vi "aryth_mux.vi"(2 "C":T1, 3 "A-B":bool, 4 "A+B":cluster{"S":bool, "C":bool}) -> (0 "R":bool, 1 "S1":bool)   [LabVIEW 2013]
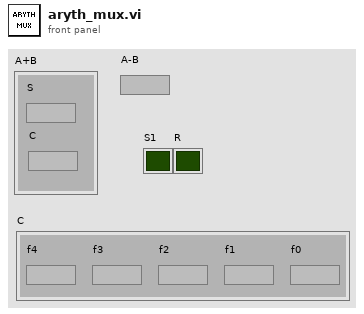
[diagram p1: front panel]
types:
  T1 = cluster{"f4":bool, "f3":bool, "f2":bool, "f1":bool, "f0":bool}
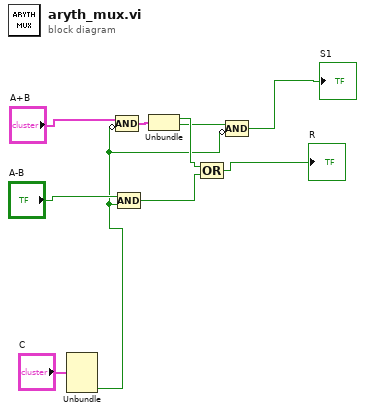
[diagram p0: block diagram]
diagram:
  n1 = Unbundle("C") -> ("f0"=w4:bool)  [unwired: 4 out]
  n2 = Compound Arithmetic op=AND("A+B", invert w4) -> (w7:cluster{"S":bool, "C":bool})
  n3 = Compound Arithmetic op=AND("A-B", w4) -> (w5:bool)
  n4 = Unbundle(w7) -> ("S"=w6:bool, "C"=w3:bool)
  n5 = Compound Arithmetic op=OR(w6, w5) -> (→"R":bool)
  n6 = Compound Arithmetic op=AND(w3, invert w4) -> (→"S1":bool)
